vi "Source V2.vi"(8 "error in":errorcluster, 9 "V2 rate":dbl, 10 "V2":dbl, 11 "VISA in":refnum<visa-resource-name>) -> (0 "error out":errorcluster, 1 "measured I":dbl, 2 "measured V":dbl, 3 "VISA out":refnum<visa-resource-name>)   [LabVIEW 2016, in "RP100.lvclass"]
uses:
  RP100.lvclass
  Typedefs/Output Channel--Enum.ctl
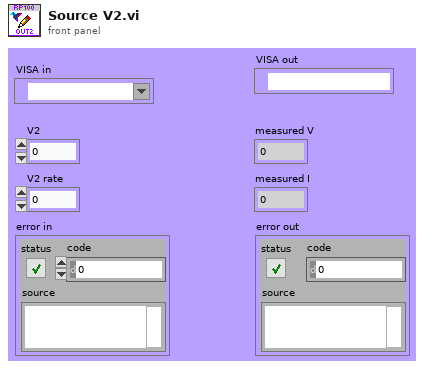
[diagram p1: front panel]
types:
  T1 = typedef "RP100.lvclass/Output Channel--Enum.ctl" = enum16{"Output 1", "Output 2"}
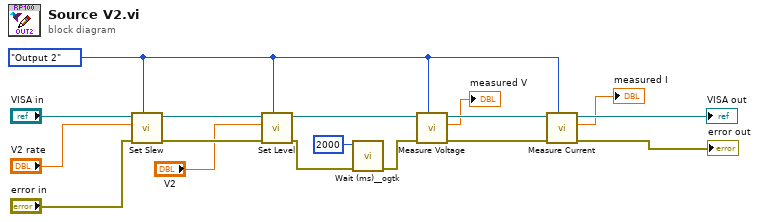
[diagram p0: block diagram]
diagram:
  w1 = Output_Channel--Enum."Output 2" ("Output")
  n1 = call "Set Slew.vi"("Output Channel"=w1, "error in (no error)"="error in", "Slew (V/s)"="V2 rate", "VISA Refnum in"="VISA in") -> ("error out"=w14:errorcluster, "VISA Refnum out"=w13:refnum<visa-resource-name>)  [unwired: 6 in]
  n2 = call "Set Level.vi"("Output Channel"=w1, "error in (no error)"=w14, "Level (V)"="V2", "VISA Refnum in"=w13) -> ("error out"=w6:errorcluster, "VISA Refnum out"=w11:refnum<visa-resource-name>)  [unwired: 6 in]
  n3 = call <userlib>:"Wait (ms)__ogtk.vi"("error in (no error)"=w6, "milliseconds to wait"=u32 2000) -> ("error out"=w5:errorcluster)  [unwired: 8 in, 1 out]
  n4 = call "Measure Voltage.vi"("Output"=w1, "error in (no error)"=w5, "VISA Refnum in"=w11) -> ("error out"=w9:errorcluster, "measured V"=→"measured V":dbl, "VISA Refnum out"=w8:refnum<visa-resource-name>)  [unwired: 6 in]
  n5 = call "Measure Current.vi"("OutputChannel"=w1, "error in (no error)"=w9, "VISA Refnum in"=w8) -> ("error out"=→"error out":errorcluster, "measured I"=→"measured I":dbl, "VISA Refnum out"=→"VISA out":refnum<visa-resource-name>)  [unwired: 6 in]
